vi "Oil_Consumption (SubVI).vi"(9 "act_b":dbl[](array[numeric]), 11 "not.Sim_Running":bool) -> (3 "Oil Consumption [L]":dbl)   [LabVIEW 2017]
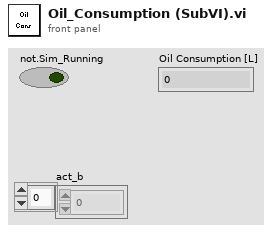
[diagram p1: front panel]
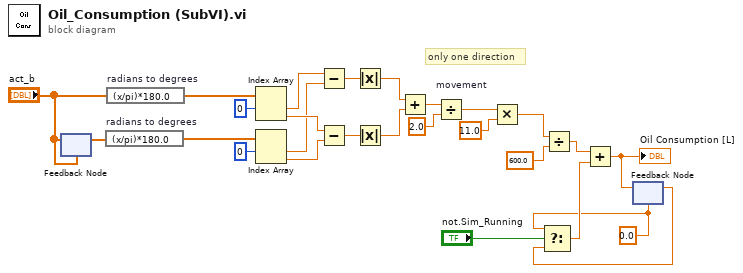
[diagram p0: block diagram]
diagram:
  w19 = 0.0 ("y")
  # "only one direction"
  n1 = feedback #1("act_b") -> (w2:dbl[])
  n2 = feedback-in #1("act_b") -> ()
  n3 = expression code="(x/pi)*180.0" "radians to degrees"(w2) -> (w23:dbl[])
  n4 = expression code="(x/pi)*180.0" "radians to degrees"("act_b") -> (w24:dbl[])
  n5 = Index Array(array=w24, index #1=0 ("index")) -> (element #1=w6:dbl, element #2=w8:dbl)  [unwired: 1 in]
  n6 = Index Array(array=w23, index #1=0 ("index")) -> (element #1=w7:dbl, element #2=w9:dbl)  [unwired: 1 in]
  n7 = Subtract(x=w6, y=w7) -> (x-y=w15:dbl)
  n8 = Subtract(x=w8, y=w9) -> (x-y=w16:dbl)
  n9 = Absolute Value(x=w15) -> (abs(x)=w10:dbl)
  n10 = Absolute Value(x=w16) -> (abs(x)=w11:dbl)
  n11 = Add(x=w10, y=w11) -> (x+y=w14:dbl)
  n12 = Divide "movement"(x=w14, y=2.0) -> (x/y=w18:dbl)
  n13 = Multiply(x=w18, y=11.0) -> (x*y=w17:dbl)
  n14 = Divide(x=w17, y=600.0) -> (x/y=w21:dbl)
  n15 = feedback #2(w19) -> (w20:dbl)
  n16 = Select(t=w19, s="not.Sim_Running", f=w20) -> (s? t:f=w22:dbl)
  n17 = Add(x=w21, y=w22) -> (x+y=w3:dbl)
  "Oil Consumption [L]" <- w3
  n18 = feedback-in #2(w3) -> ()
